vi "Cancel Notification.vi"(8 "error in":errorcluster, 11 "NotifierMessageTransport in":refnum<class "NotifierMessageTransport.lvclass">) -> (0 "error out":errorcluster, 3 "NotifierMessageTransport out":refnum<class "NotifierMessageTransport.lvclass">)   [LabVIEW 2016, in "NotifierMessageTransport.lvclass"]
uses:
  NotifierMessageTransport.lvclass
  IMessagePayload/IMessagePayload.lvclass
  NotifierMessageTransport.lvclass/NotifierMessageTransport.ctl
panel:
  out "Canceled Notification":refnum<class "IMessagePayload.lvclass">
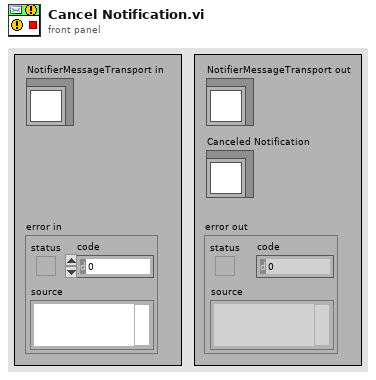
[diagram p1: front panel]
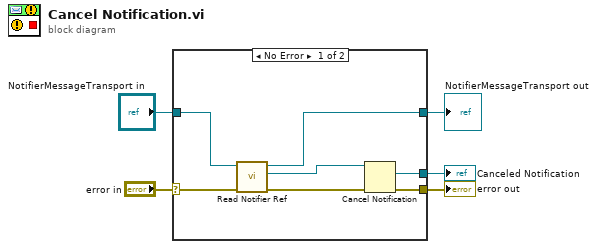
[diagram p0: block diagram]
diagram:
  n1 = case shown="No Error" "error in" {
    selector: "error in" -> [w9 w14]
    tunnel: [w7 w14] -> w4
    tunnel: [w11 w13] -> w2
    tunnel: "NotifierMessageTransport in" -> [w12 w13]
    tunnel: [w6 _] -> w1
    frame No Error {
      n2 = call "Read Notifier Ref.vi"("error in"=w9, "NotifierMessageTransport in"=w12) -> ("error out"=w10:errorcluster, "Notifier Ref"=w8:refnum<notifier>, "NotifierMessageTransport out"=w11:refnum<class "NotifierMessageTransport.lvclass">)  [unwired: 7 in]
      n3 = Cancel Notification(0:w8, 3:w10) -> (9:w6:refnum<class "IMessagePayload.lvclass">, 11:w7:errorcluster)  [unwired: 1 out]
    }
    frame Error {
    }
  }
  "error out" <- w4
  "NotifierMessageTransport out" <- w2
  "Canceled Notification" <- w1
